vi "VPConv_SM.vi"() -> ()   [LabVIEW 2019]
uses:
  <vilib>/Utility/file.llb/Write Delimited Spreadsheet (DBL).vi
  <vilib>/Utility/file.llb/Read Delimited Spreadsheet (DBL).vi
  <vilib>/Analysis/NI_AALBase.lvlib
panel:
  out "Current State":string
  in  "Tab Control":enum32{"Mask A", "Mask B"}(tab)
  out "Intensity A":cluster{dbl[], dbl[]}[](graph)
  out "Phase A":cluster{"Ramp Pattern":dbl[], "phase out":dbl[]}(graph)
  out "Cur A":sgl
  out "Intensity B":cluster{dbl[], dbl[]}[](graph)
  out "Phase B":cluster{"Ramp Pattern":dbl[], "phase out":dbl[]}(graph)
  out "Cur B":sgl
  in  "Use Max Voltage Range for B?":bool
  in  "Save Path":path=path "C:/Users/Pubudu Wijesinghe/Desktop/VPConv"
  in  "Calib Path":path=path "C:/Users/Pubudu Wijesinghe/Desktop/Voltage Calib"
  in  "Min Cut-off":sgl=0.25
  in  "Max Cut-on":sgl=0.75
  in  "Ending Pixel":sgl=500.0
  in  "Starting Pixel":sgl=200.0
  in  "Use Max Voltage Range for A?":bool
  in  "OK":bool
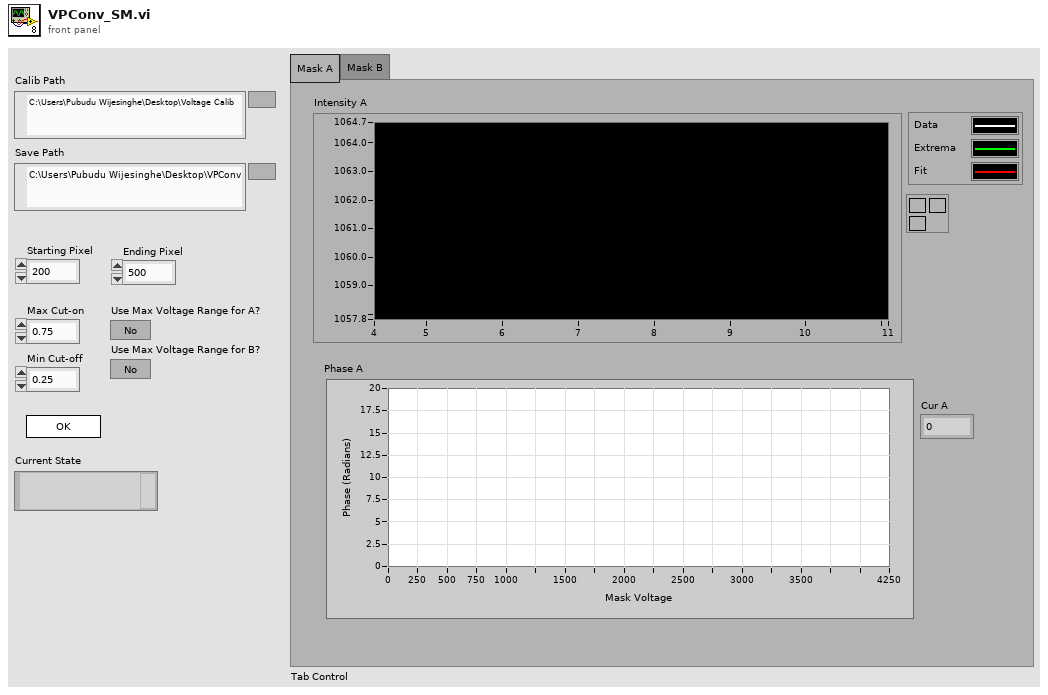
[diagram p1: front panel]
types:
  T1 = enum32{"Invalid", "Standard", "Closed", "Hidden", "Minimized", "Maximized"}
  T2 = enum32{"invalid app kind", "Development System", "Run Time System", "Student Edition", "Embedded LabVIEW", "Evaluation", "Custom"}
  T3 = cluster{"Core":cluster{"Current VI Reference":refnum<vi>, "Close Panel on Exit?":bool}, "Your Boolean data":bool, "Your string data":string, "Calib Path":path, "Save Path":path, "Starting Pixel":sgl, "Ending Pixel":sgl, "Max Cut-on":sgl, "Min Cut-off":sgl}
  T4 = cluster{"Current VI Reference":refnum<vi>, "Close Panel on Exit?":bool}
  T5 = cluster{"type":enum16{"minimum", "maximum"}, "x":i32, "y":dbl}[]
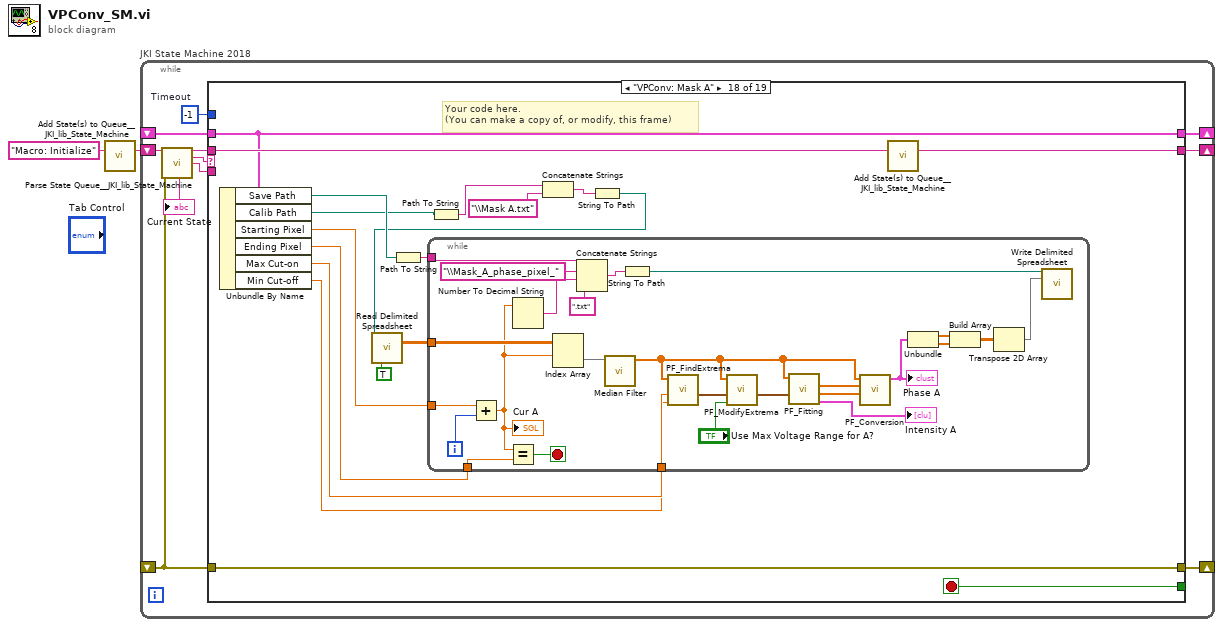
[diagram p0: block diagram]
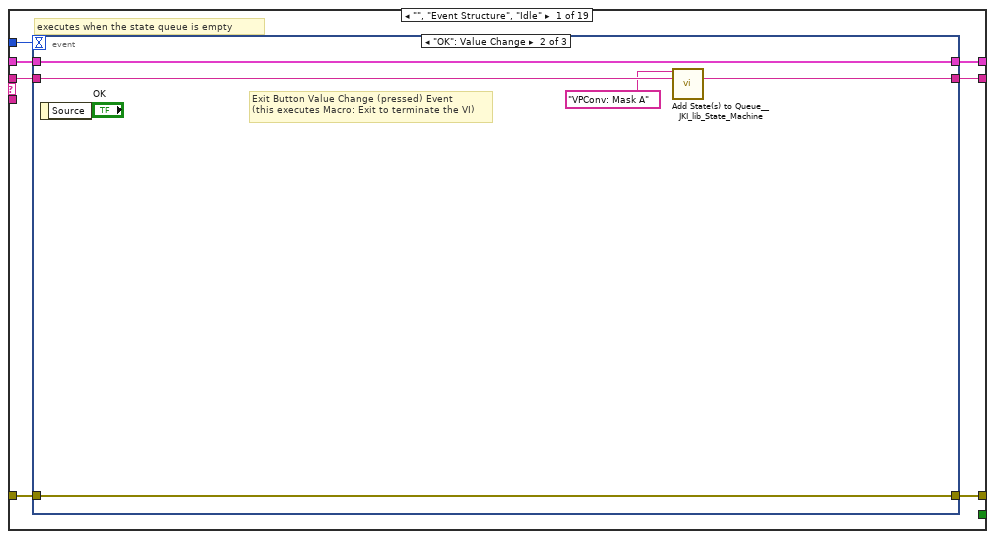
[diagram p2: hidden frame]
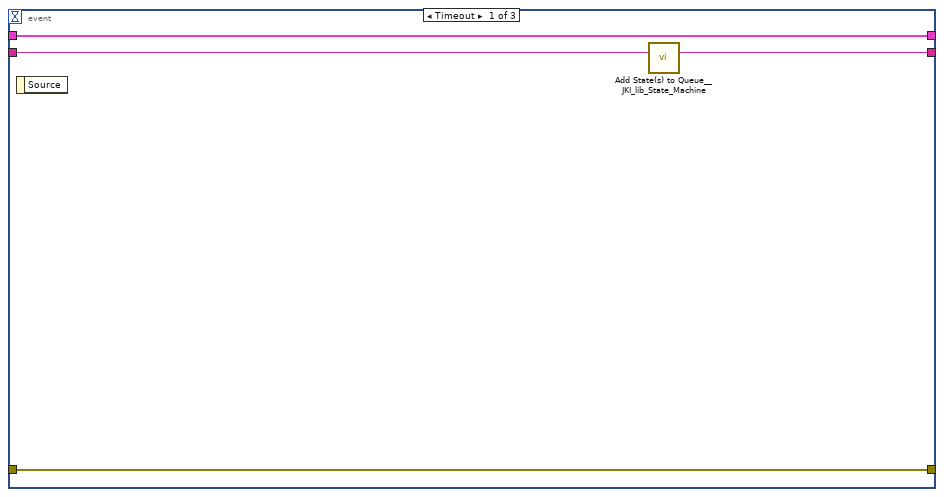
[diagram p3: hidden frame]
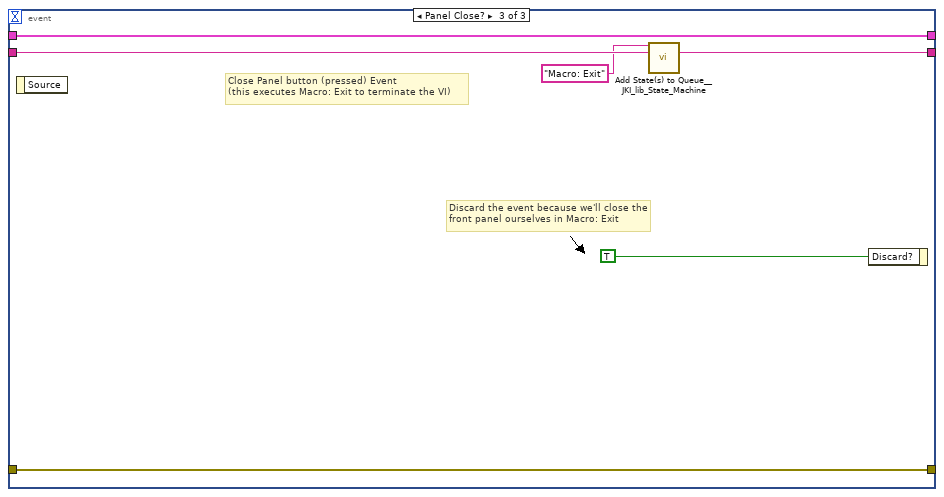
[diagram p4: hidden frame]
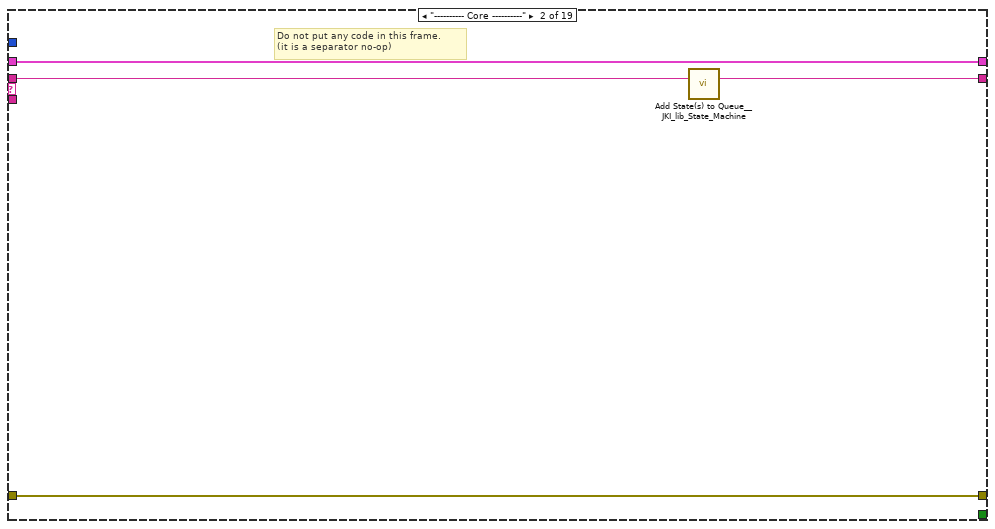
[diagram p5: hidden frame]
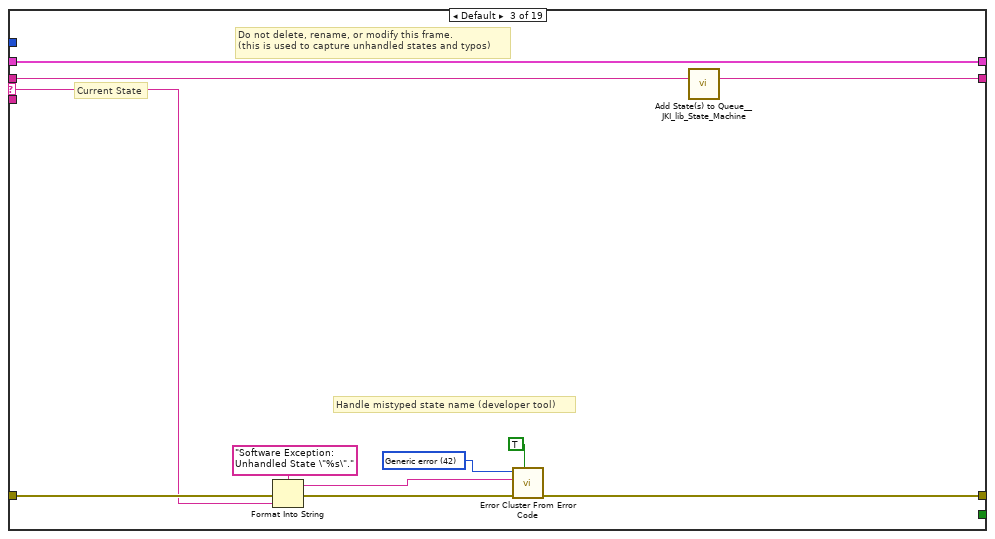
[diagram p6: hidden frame]
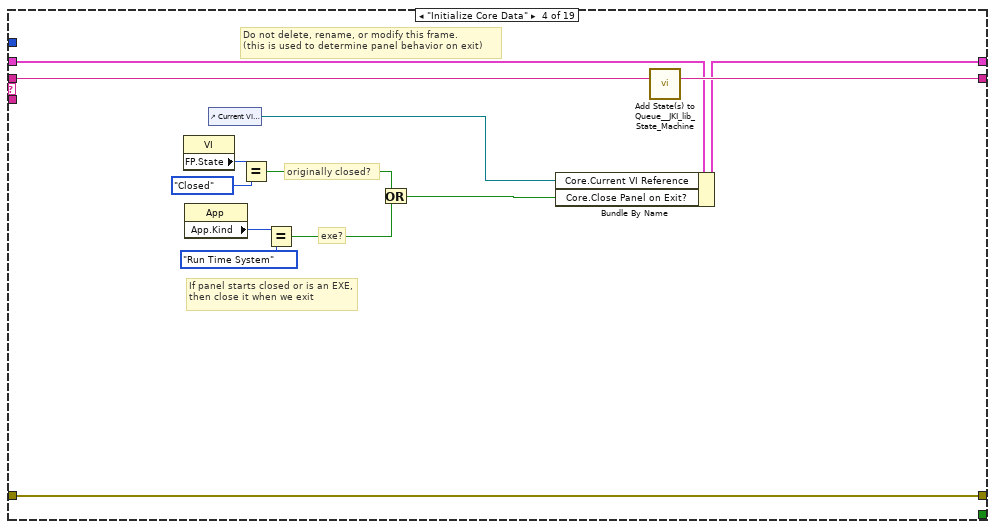
[diagram p7: hidden frame]
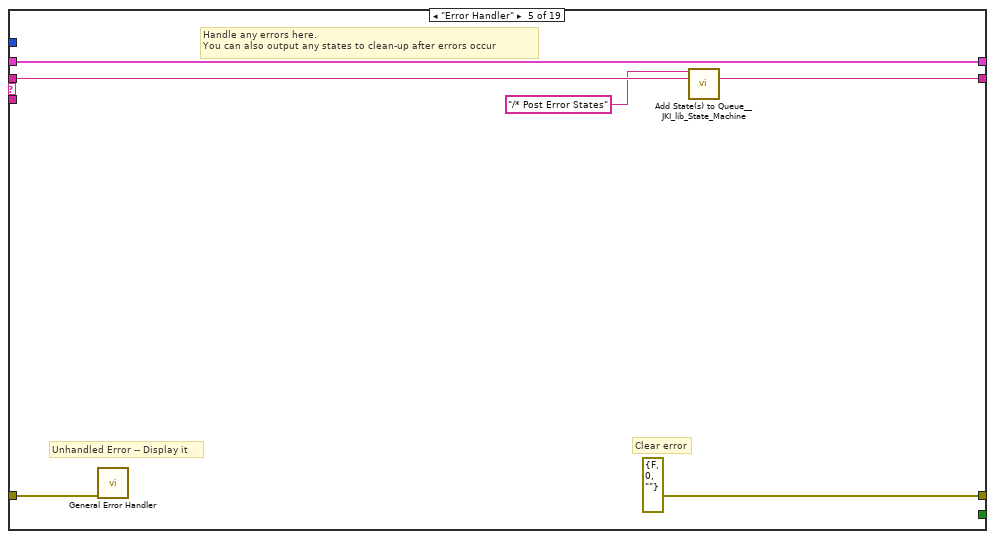
[diagram p8: hidden frame]
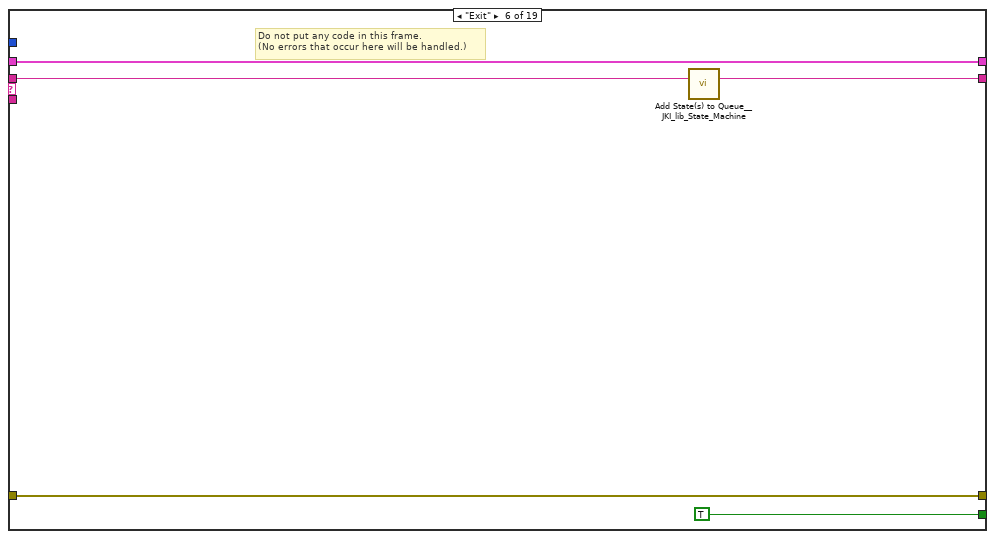
[diagram p9: hidden frame]
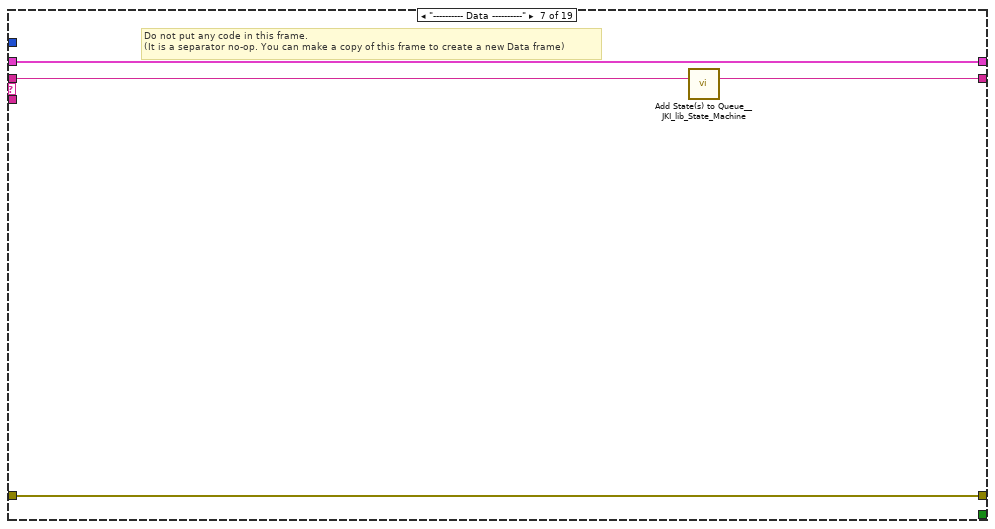
[diagram p10: hidden frame]
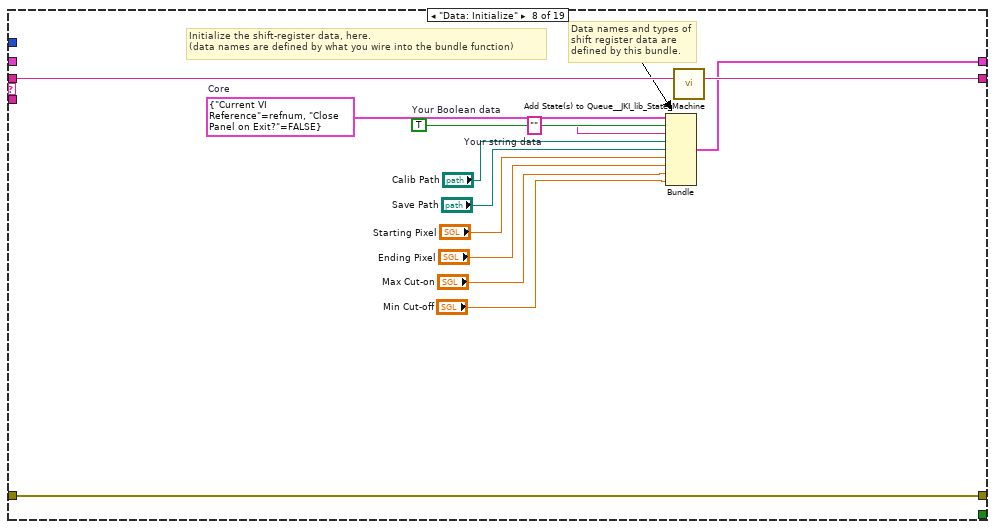
[diagram p11: hidden frame]
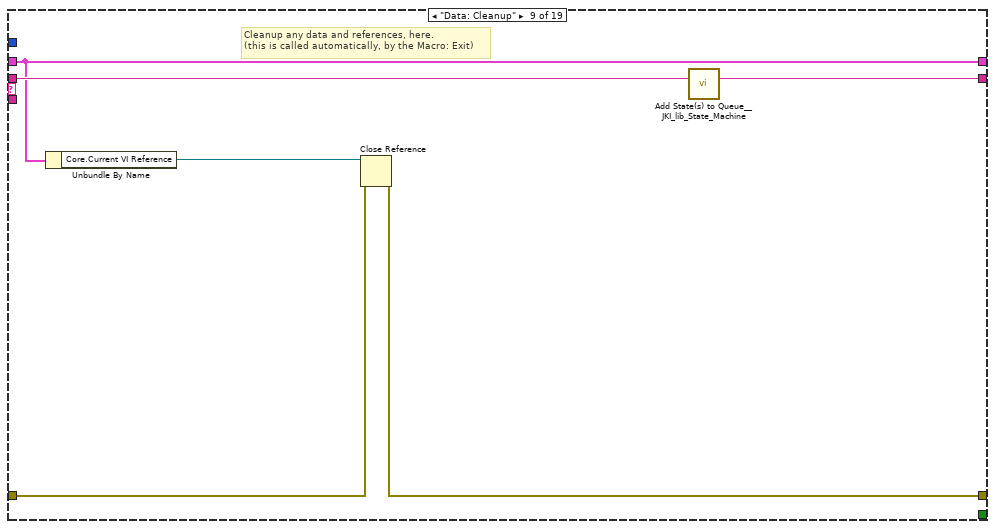
[diagram p12: hidden frame]
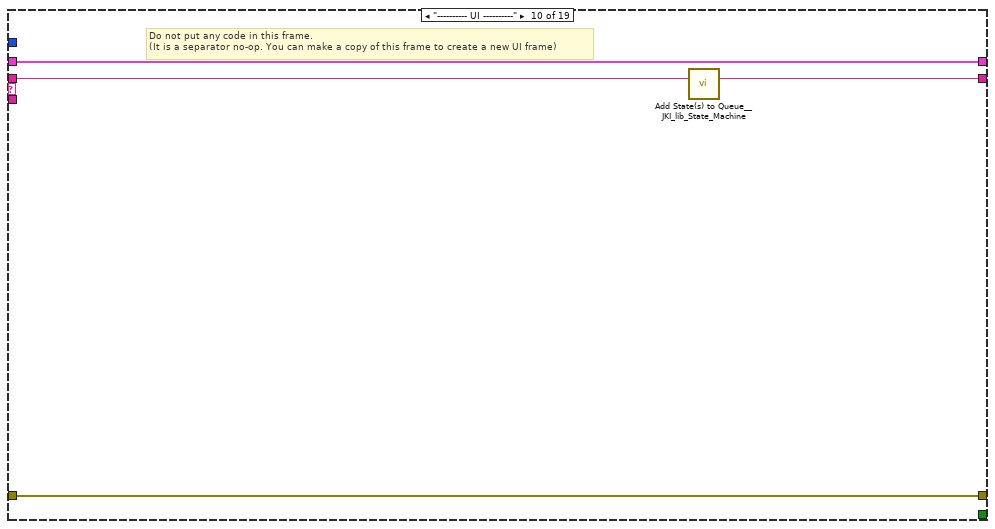
[diagram p13: hidden frame]
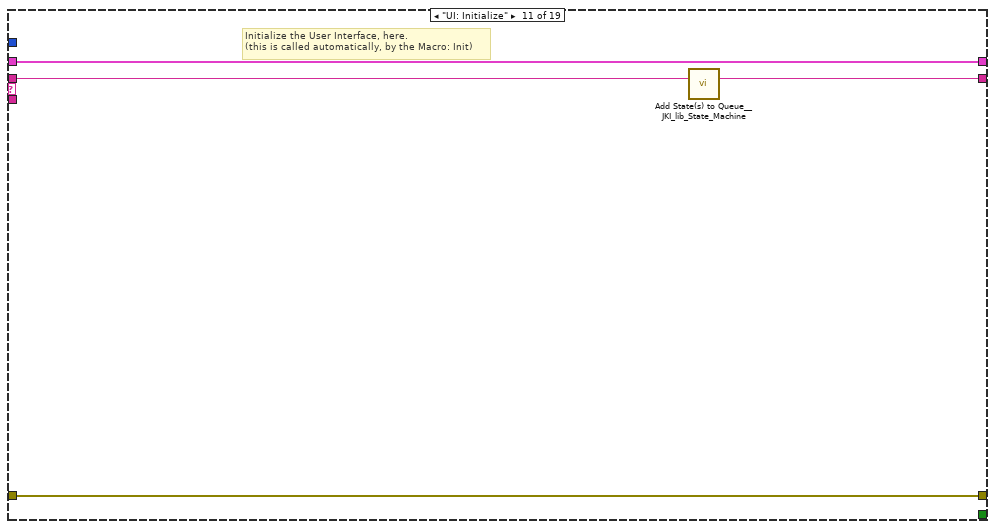
[diagram p14: hidden frame]
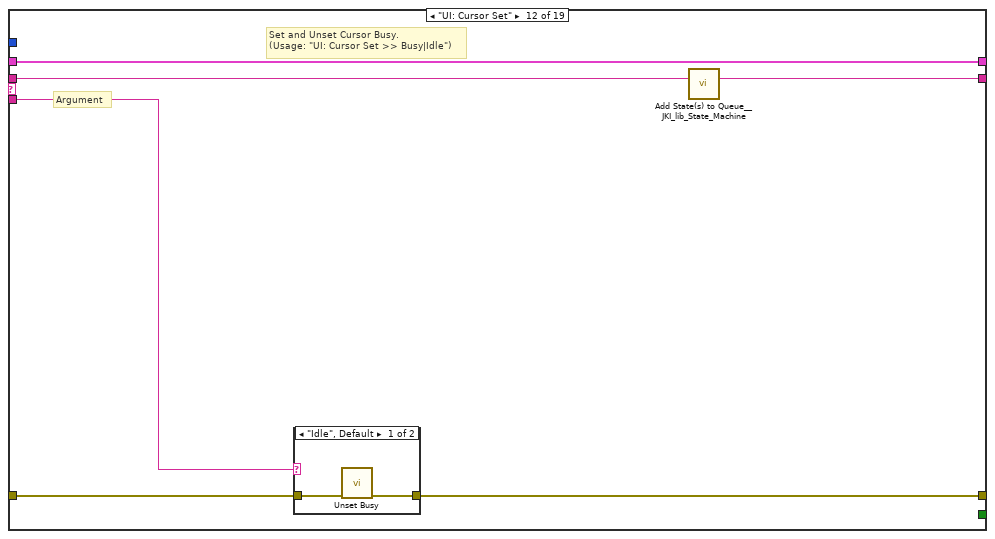
[diagram p15: hidden frame]
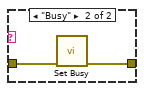
[diagram p16: hidden frame]
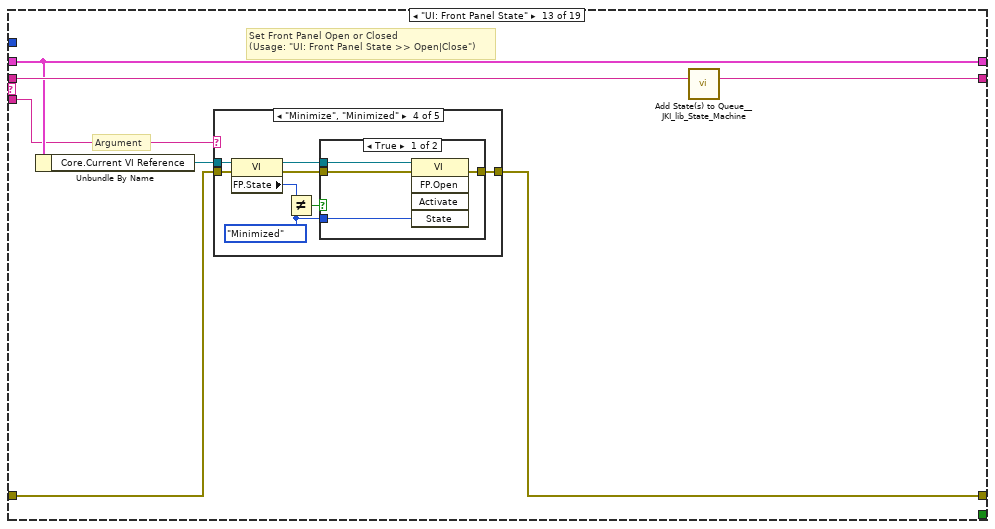
[diagram p17: hidden frame]
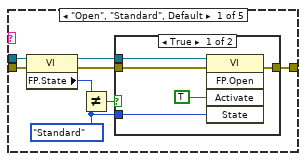
[diagram p18: hidden frame]
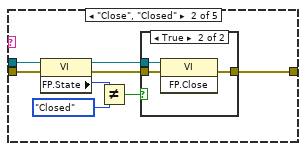
[diagram p20: hidden frame]
diagram:
  n1 = call <vilib>:"Add State(s) to Queue__JKI_lib_State_Machine.vi"("State(s) in (\"\")"="Macro: Initialize") -> ("States Out"=w2:string)  [unwired: 14 in]
  n2 = while "JKI State Machine 2018" {
    shift-right: [w6] -> _
    shift-left: _ -> [w5]
    shift-right: [w9] -> _
    shift-left: _ -> [w3]
    shift-right: [w8] -> _
    shift-left: w2 -> [w10]
    stop <- w7 stop-if-true
    w4 = -1  # Timeout
    n3 = call <vilib>:"Parse State Queue__JKI_lib_State_Machine.vi"("State Queue"=w10, "Error In (no error)"=w3) -> ("Remaining States"=w12:string, "Current State"=w13:string, "Arguments"=w11:string)  [unwired: 11 in]
    "Current State" <- w13
    n4 = case shown="\"VPConv: Mask A\"" w13 {
      selector: w13 -> [_ _ w40 _ _ _ _ _ _ _ _ _ _ _ _ _ _ _ _]
      tunnel: w12 -> [w20 w39 w44 w63 w69 w74 w78 w91 w97 w101 w105 w111 w122 w191 w196 w206 w210 w227 w271]
      tunnel: w11 -> [_ _ _ _ _ _ _ _ _ _ _ w106 w116 _ _ _ _ _ _]
      tunnel: w5 -> [w18 w36 w42 w56 w66 w72 w75 _ w92 w98 w103 w109 w118 w188 w193 w203 w207 w222 w266]
      tunnel: [w17 w37 w46 w60 errorcluster {"status"=FALSE, "code"=0, "source"=""} ("error out") w71 w76 w88 w93 w99 w102 w107 w119 w189 w194 w204 w208 w225 w269] -> w9
      tunnel: w3 -> [w16 w37 w45 w60 w65 w71 w76 w88 w94 w99 w102 w108 w120 w189 w194 w204 w208 w225 w269]
      tunnel: [w19 w38 w43 w62 w68 w73 w77 w90 w96 w100 w104 w110 w121 w190 w195 w205 w209 w226 w270] -> w8
      tunnel: [_ _ _ _ _ TRUE _ _ _ _ _ _ _ _ _ _ _ _ _] -> w7
      tunnel: [w15 w36 w42 w61 w66 w72 w75 w89 w92 w98 w103 w109 w118 w188 w193 w203 w207 w222 w266] -> w6
      tunnel: w4 -> [w14 _ _ _ _ _ _ _ _ _ _ _ _ _ _ _ _ _ _]
      frame "", "Event Structure", "Idle" {
        # "executes when the state queue is empty"
        n5 = event shown="[1] \"OK\": Value Change" {
          selector: _ -> [_ _ _]
          dyn-events: _ -> [_ _ _]
          timeout: w14 -> [_ _ _]
          tunnel: w20 -> [w24 w29 w35]
          tunnel: [w23 w28 w34] -> w19
          tunnel: w18 -> [w21 w26 w32]
          tunnel: [w22 w27 w33] -> w17
          tunnel: w16 -> [w22 w27 w33]
          tunnel: [w21 w26 w32] -> w15
          event Timeout {
            n6 = event-data() -> ()  [unwired: 1 in, 1 out]
            n7 = call <vilib>:"Add State(s) to Queue__JKI_lib_State_Machine.vi"("State(s) in (\"\")"=w24) -> ("States Out"=w23:string)  [unwired: 14 in]
          }
          event "OK": Value Change {
            # "Exit Button Value Change (pressed) Event\n(this executes Macro: Exit to terminate the VI)"
            n8 = event-data() -> ()  [unwired: 1 in, 1 out]
            n9 = call <vilib>:"Add State(s) to Queue__JKI_lib_State_Machine.vi"("State(s) in Front (\"\")"="VPConv: Mask A", "State(s) in (\"\")"=w29) -> ("States Out"=w28:string)  [unwired: 13 in]
          }
          event Panel Close? {
            # "Discard the event because we'll close the front panel ourselves in Macro: Exit"
            # "Close Panel button (pressed) Event\n(this executes Macro: Exit to terminate the VI)"
            n10 = event-data() -> ()  [unwired: 1 in, 1 out]
            n11 = call <vilib>:"Add State(s) to Queue__JKI_lib_State_Machine.vi"("State(s) in Front (\"\")"="Macro: Exit", "State(s) in (\"\")"=w35) -> ("States Out"=w34:string)  [unwired: 13 in]
            n12 = event-data("Discard?"=TRUE) -> ()  [unwired: 1 in, 1 out]
          }
        }
      }
      frame "---------- Core ----------" {
        # "Do not put any code in this frame.\n(it is a separator no-op)"
        n13 = call <vilib>:"Add State(s) to Queue__JKI_lib_State_Machine.vi"("State(s) in (\"\")"=w39) -> ("States Out"=w38:string)  [unwired: 14 in]
      }
      frame Default {
        w49 = 42 items=["No error", "Argument error", "Memory is full", "Out of zone", "End of file", "File already open", "Generic file I/O error", "File not found", "File permission error", "Disk is full", "Duplicate path", "Too many files open", "System feature not enabled", "Resource file not found", "Cannot add resource", "Resource not found", "Image not found", "Image memory error", "Pen does not exist", "Config type invalid", "Config token not found", "Config parse error", "Config memory error", "Bad external code format", "Bad external code offset", "External code not present", "Null window", "Destroy window error", "Null menu", "Print aborted", "Bad print record", "Print driver error", "Windows error during printing", "Memory error during printing", "Print dialog error", "Generic print error", "Invalid device refnum", "Device not found", "Device parameter error", "Device unit error", "Cannot open device", "Device call aborted", "Generic error", "Cancelled by user", "Object ID too low", "Object ID too high", "Object not in heap", "Unknown heap", "Unknown object (invalid DefProc)", "Unknown object (DefProc not in table)", "Message out of range", "Invalid (null) method", "Unknown message", "Manager call not supported", "Bad address", "Network operation in progress", "Network operation timed out", "Connection is busy", "Network attribute not supported", "Network error", "Address in use", "System out of memory", "Connection aborted", "Connection refused", "Not connected", "Already connected", "Connection closed", "Initialization error (interapplication manager)", "Bad occurrence", "Wait on unbound occurrence handler", "Occurrence queue overflow", "Datalog type conflict", "Unused", "Unrecognized type (interapplication manager)", "Memory corrupt", "Failed to make temporary DLL", "Old CIN version", "Drag socket not found", "Failed to load drop-object", "Failed to register OLE object", "Failed to release OLE object", "Format specifier type mismatch", "Unknown format specifier", "Too few format specifiers", "Too many format specifiers", "Scan failed", "Newer CIN version", "Error converting to variant", "Runtime menu error", "Password tampered", "Variant attribute not found", "Incompatible variant data type", "Event data is not available", "Event Store is not present", "Occurrence is not found", "Event Queue is not created", "Event info is not available", "Refnum passed is NULL", "Error retrieving Class GUID", "Error retrieving CoClass GUID", "Error retrieving TypeLib GUID.", "Bad built application magic bytes.", "Specific driver is different from the specific driver associated with the Logical Name.", "There is no session opened to the class driver.", "Max Error", "MAX - Error with config objects", "MAX - Error loading configuration", "MAX - Group not supported"]
        # "Current State"
        # "Do not delete, rename, or modify this frame.\n(this is used to capture unhandled states and typos)"
        # "Handle mistyped state name (developer tool)"
        n14 = Format Into String(format string="Software Exception: Unhandled State \"%s\"." ("message"), error in=w45, w40) -> (resulting string=w48:string, error out=w47:errorcluster)  [unwired: 1 in]
        n15 = call <vilib>:"Error Cluster From Error Code.vi"("show call chain? (False)"=TRUE, "error in (no error)"=w47, "error message (\"\")"=w48, "error code (0)"=w49) -> ("error out"=w46:errorcluster)  [unwired: 5 in]
        n16 = call <vilib>:"Add State(s) to Queue__JKI_lib_State_Machine.vi"("State(s) in (\"\")"=w44) -> ("States Out"=w43:string)  [unwired: 14 in]
      }
      frame "Initialize Core Data" {
        # "Do not delete, rename, or modify this frame.\n(this is used to determine panel behavior on exit)"
        # "originally closed?"
        # "exe?"
        # "If panel starts closed or is an EXE, then close it when we exit"
        n17 = property class="VI"() -> ("FP.State"=w53:T1)  [unwired: 2 in, 2 out]
        n18 = property class="App"() -> ("App.Kind"=w59:T2)  [unwired: 2 in, 2 out]
        n19 = control-ref of="Current VI Reference"() -> (w54:refnum<vi>)
        n20 = Equal?(x=w53, y=T1."Closed" ("Front Panel Window:State")) -> (x = y?=w51:bool)
        n21 = Equal?(x=w59, y=T2."Run Time System" ("Application:Kind")) -> (x = y?=w57:bool)
        n22 = Or(x=w51, y=w57) -> (x .or. y?=w55:bool)
        n23 = Bundle By Name(cluster=w56, "Core.Current VI Reference"=w54, "Core.Close Panel on Exit?"=w55) -> (w61:T3)
        n24 = call <vilib>:"Add State(s) to Queue__JKI_lib_State_Machine.vi"("State(s) in (\"\")"=w63) -> ("States Out"=w62:string)  [unwired: 14 in]
      }
      frame "Error Handler" {
        # "Unhandled Error -- Display it"
        # "Handle any errors here.\nYou can also output any states to clean-up after errors occur"
        # "Clear error"
        n25 = call <vilib>:"General Error Handler.vi"("error in (no error)"=w65) -> ()  [unwired: 10 in, 5 out]
        n26 = call <vilib>:"Add State(s) to Queue__JKI_lib_State_Machine.vi"("State(s) in Front (\"\")"="/* Post Error States", "State(s) in (\"\")"=w69) -> ("States Out"=w68:string)  [unwired: 13 in]
      }
      frame "Exit" {
        # "Do not put any code in this frame.\n(No errors that occur here will be handled.)"
        n27 = call <vilib>:"Add State(s) to Queue__JKI_lib_State_Machine.vi"("State(s) in (\"\")"=w74) -> ("States Out"=w73:string)  [unwired: 14 in]
      }
      frame "---------- Data ----------" {
        # "Do not put any code in this frame.\n(It is a separator no-op. You can make a copy of this frame to create a new Data frame)"
        n28 = call <vilib>:"Add State(s) to Queue__JKI_lib_State_Machine.vi"("State(s) in (\"\")"=w78) -> ("States Out"=w77:string)  [unwired: 14 in]
      }
      frame "Data: Initialize" {
        w85 = T4 {"Current VI Reference"=refnum, "Close Panel on Exit?"=FALSE}  # Core
        w87 = TRUE  # Your Boolean data
        w86 = ""  # Your string data
        # "Data names and types of shift register data are defined by this bundle."
        # "Initialize the shift-register data, here.\n(data names are defined by what you wire into the bundle function)"
        n29 = Bundle("Core"=w85, "Your Boolean data"=w87, "Your string data"=w86, "Calib Path"="Calib Path", "Save Path"="Save Path", "Starting Pixel"="Starting Pixel", "Ending Pixel"="Ending Pixel", "Max Cut-on"="Max Cut-on", "Min Cut-off"="Min Cut-off") -> (w89:T3)  [unwired: 1 in]
        n30 = call <vilib>:"Add State(s) to Queue__JKI_lib_State_Machine.vi"("State(s) in (\"\")"=w91) -> ("States Out"=w90:string)  [unwired: 14 in]
      }
      frame "Data: Cleanup" {
        # "Cleanup any data and references, here.\n(this is called automatically, by the Macro: Exit)"
        n31 = Unbundle By Name(w92) -> ("Core.Current VI Reference"=w95:refnum<vi>)
        n32 = Close Reference(reference=w95, error in (no error)=w94) -> (error out=w93:errorcluster)
        n33 = call <vilib>:"Add State(s) to Queue__JKI_lib_State_Machine.vi"("State(s) in (\"\")"=w97) -> ("States Out"=w96:string)  [unwired: 14 in]
      }
      frame "---------- UI ----------" {
        # "Do not put any code in this frame.\n(It is a separator no-op. You can make a copy of this frame to create a new UI frame)"
        n34 = call <vilib>:"Add State(s) to Queue__JKI_lib_State_Machine.vi"("State(s) in (\"\")"=w101) -> ("States Out"=w100:string)  [unwired: 14 in]
      }
      frame "UI: Initialize" {
        # "Initialize the User Interface, here.\n(this is called automatically, by the Macro: Init)"
        n35 = call <vilib>:"Add State(s) to Queue__JKI_lib_State_Machine.vi"("State(s) in (\"\")"=w105) -> ("States Out"=w104:string)  [unwired: 14 in]
      }
      frame "UI: Cursor Set" {
        # "Argument"
        # "Set and Unset Cursor Busy.\n(Usage: \"UI: Cursor Set >> Busy|Idle\")"
        n36 = case shown="\"Idle\", Default" w106 {
          tunnel: w108 -> [w113 w115]
          tunnel: [w112 w114] -> w107
          frame "Idle", Default {
            n37 = call <vilib>:"Unset Busy.vi"("error in (no error)"=w113) -> ("error out"=w112:errorcluster)  [unwired: 10 in]
          }
          frame "Busy" {
            n38 = call <vilib>:"Set Busy.vi"("error in (no error)"=w115) -> ("error out"=w114:errorcluster)  [unwired: 9 in, 1 out]
          }
        }
        n39 = call <vilib>:"Add State(s) to Queue__JKI_lib_State_Machine.vi"("State(s) in (\"\")"=w111) -> ("States Out"=w110:string)  [unwired: 14 in]
      }
      frame "UI: Front Panel State" {
        # "Argument"
        # "Set Front Panel Open or Closed\n(Usage: \"UI: Front Panel State >> Open|Close\")"
        n40 = Unbundle By Name(w118) -> ("Core.Current VI Reference"=w117:refnum<vi>)
        n41 = case shown="\"Minimize\", \"Minimized\"" w116 {
          tunnel: w120 -> [w128 w143 w154 w167 w180]
          tunnel: [w130 w144 w156 w169 w182] -> w119
          tunnel: w117 -> [w129 w141 w155 w168 w181]
          frame "Open", "Standard", Default {
            w123 = T1."Standard" ("State")
            n42 = property class="VI"(reference=w129, error in=w128) -> (reference out=w126:refnum<vi>, error out=w127:errorcluster, "FP.State"=w125:T1)
            n43 = Not Equal?(x=w125, y=w123) -> (x != y?=w124:bool)
            n44 = case shown="True" w124 {
              tunnel: [w134 w136] -> w130
              tunnel: w127 -> [w133 w136]
              tunnel: w126 -> [w132 _]
              tunnel: w123 -> [w131 _]
              frame True {
                n45 = invoke class="VI" method="FP.Open"(reference=w132, error in=w133, "Activate"=TRUE, "State"=w131) -> (error out=w134:errorcluster)  [unwired: 1 in, 4 out]
              }
              frame False {
              }
            }
          }
          frame "Close", "Closed" {
            n46 = property class="VI"(reference=w141, error in=w143) -> (reference out=w140:refnum<vi>, error out=w142:errorcluster, "FP.State"=w138:T1)
            n47 = Not Equal?(x=w138, y=T1."Closed" ("Front Panel Window:State")) -> (x != y?=w137:bool)
            n48 = case shown="True" w137 {
              tunnel: [w145 w148] -> w144
              tunnel: w142 -> [w145 w147]
              tunnel: w140 -> [_ w146]
              frame False {
              }
              frame True {
                n49 = invoke class="VI" method="FP.Close"(reference=w146, error in=w147) -> (error out=w148:errorcluster)  [unwired: 1 in, 2 out]
              }
            }
          }
          frame "Hidden", "Hide" {
            w149 = T1."Hidden" ("State")
            n50 = property class="VI"(reference=w155, error in=w154) -> (reference out=w152:refnum<vi>, error out=w153:errorcluster, "FP.State"=w151:T1)
            n51 = Not Equal?(x=w151, y=w149) -> (x != y?=w150:bool)
            n52 = case shown="True" w150 {
              tunnel: [w160 w161] -> w156
              tunnel: w153 -> [w159 w161]
              tunnel: w152 -> [w158 _]
              tunnel: w149 -> [w157 _]
              frame True {
                n53 = invoke class="VI" method="FP.Open"(reference=w158, error in=w159, "State"=w157) -> (error out=w160:errorcluster)  [unwired: 2 in, 4 out]
              }
              frame False {
              }
            }
          }
          frame "Minimize", "Minimized" {
            w162 = T1."Minimized" ("State")
            n54 = property class="VI"(reference=w168, error in=w167) -> (reference out=w165:refnum<vi>, error out=w166:errorcluster, "FP.State"=w164:T1)
            n55 = Not Equal?(x=w164, y=w162) -> (x != y?=w163:bool)
            n56 = case shown="True" w163 {
              tunnel: [w173 w174] -> w169
              tunnel: w166 -> [w172 w174]
              tunnel: w165 -> [w171 _]
              tunnel: w162 -> [w170 _]
              frame True {
                n57 = invoke class="VI" method="FP.Open"(reference=w171, error in=w172, "State"=w170) -> (error out=w173:errorcluster)  [unwired: 2 in, 4 out]
              }
              frame False {
              }
            }
          }
          frame "Maximize", "Maximized" {
            w175 = T1."Maximized" ("State")
            n58 = property class="VI"(reference=w181, error in=w180) -> (reference out=w178:refnum<vi>, error out=w179:errorcluster, "FP.State"=w177:T1)
            n59 = Not Equal?(x=w177, y=w175) -> (x != y?=w176:bool)
            n60 = case shown="True" w176 {
              tunnel: [w186 w187] -> w182
              tunnel: w179 -> [w185 w187]
              tunnel: w178 -> [w184 _]
              tunnel: w175 -> [w183 _]
              frame True {
                n61 = invoke class="VI" method="FP.Open"(reference=w184, error in=w185, "State"=w183) -> (error out=w186:errorcluster)  [unwired: 2 in, 4 out]
              }
              frame False {
              }
            }
          }
        }
        n62 = call <vilib>:"Add State(s) to Queue__JKI_lib_State_Machine.vi"("State(s) in (\"\")"=w122) -> ("States Out"=w121:string)  [unwired: 14 in]
      }
      frame "---------- Macro ----------" {
        # "Do not put any code in this frame.\n(It is a separator no-op. You can make a copy of this frame to create a new Macro frame)"
        n63 = call <vilib>:"Add State(s) to Queue__JKI_lib_State_Machine.vi"("State(s) in (\"\")"=w191) -> ("States Out"=w190:string)  [unwired: 14 in]
      }
      frame "Macro: Initialize" {
        w192 = "Data: Initialize\nInitialize Core Data\nUI: Initialize\nUI: Front Panel State >> Open"  # Data: Initialize Initialize Core Data UI: Initialize UI: Front Panel State >> Open
        # "Initialization Macro\n(This is called once, when the VI starts)"
        n64 = call <vilib>:"Add State(s) to Queue__JKI_lib_State_Machine.vi"("State(s) in Front (\"\")"=w192, "State(s) in (\"\")"=w196) -> ("States Out"=w195:string)  [unwired: 13 in]
      }
      frame "Macro: Exit" {
        # "Exit Macro\n(This is called once, when the VI exits)"
        n65 = Unbundle By Name(w203) -> ("Core.Close Panel on Exit?"=w202:bool)
        n66 = Select(t="UI: Front Panel State >> Close", s=w202, f="") -> (s? t:f=w199:string)
        n67 = call <vilib>:"Add State(s) to Queue__JKI_lib_State_Machine.vi"("State(s) in (\"\")"=w199, "State(s) at Back (\"\")"="Data: Cleanup\nExit") -> ("States Out"=w197:string)  [unwired: 13 in]
        n68 = call <vilib>:"Add State(s) to Queue__JKI_lib_State_Machine.vi"("State(s) in Front (\"\")"=w197, "State(s) in (\"\")"=w206) -> ("States Out"=w205:string)  [unwired: 13 in]
      }
      frame "---------- VPConv ----------" {
        # "Template Separator\n(You can make a copy of, or modify, this frame)"
        n69 = call <vilib>:"Add State(s) to Queue__JKI_lib_State_Machine.vi"("State(s) in (\"\")"=w210) -> ("States Out"=w209:string)  [unwired: 14 in]
      }
      frame "VPConv: Mask A" {
        # "Your code here.\n(You can make a copy of, or modify, this frame)"
        n70 = Unbundle By Name(w222) -> ("Save Path"=w221:path, "Calib Path"=w212:path, "Starting Pixel"=w219:sgl, "Ending Pixel"=w218:sgl, "Max Cut-on"=w217:sgl, "Min Cut-off"=w216:sgl)
        n71 = Path To String(path=w221) -> (string=w220:string)
        n72 = Path To String(path=w212) -> (string=w215:string)
        n73 = Concatenate Strings(w215, "\\Mask A.txt" ("string")) -> (w213:string)
        n74 = String To Path(string=w213) -> (path=w211:path)
        n75 = call-poly <vilib>:"Read Delimited Spreadsheet.vi"("file path (dialog if empty)"=w211, "transpose? (F)"=TRUE) -> ("all rows"=w223:dbl[][])  [unwired: 8 in, 5 out]
        n76 = while {
          tunnel: w223 -> [w248]
          tunnel: w220 -> [w235]
          tunnel: w219 -> [w234]
          tunnel: w218 -> [w233]
          tunnel: w217 -> [w232]
          tunnel: w216 -> [w231]
          i -> [w246]
          stop <- w247 stop-if-true
          n77 = Add(x=w234, y=w246) -> (x+y=w243:sgl)
          "Cur A" <- w243
          n78 = Equal?(x=w243, y=w233) -> (x = y?=w247:bool)
          n79 = Number To Decimal String(number=w243) -> (decimal integer string=w244:string)  [unwired: 1 in]
          n80 = Index Array(array=w248, index (row)=w243) -> (element=w229:dbl[])  [unwired: 1 in]
          n81 = Concatenate Strings(w235, "\\Mask_A_phase_pixel_", w244, ".txt" ("string")) -> (w242:string)
          n82 = call <vilib>:"Median Filter.vi"("X"=w229) -> ("Filtered X"=w228:dbl[])  [unwired: 9 in, 1 out]
          n83 = String To Path(string=w242) -> (path=w236:path)
          n84 = call "PF_FindExtrema.vi"("Min Cut-off"=w231, "Max Cut-on"=w232, "Intensity Array"=w228) -> ("Extrema Array"=w254:T5)  [unwired: 7 in]
          n85 = call "PF_ModifyExtrema.vi"("Max Voltage Range?"="Use Max Voltage Range for A?", "Extremas Array In"=w254, "Intensity Array"=w228) -> ("Extremas Array Out"=w252:T5)  [unwired: 8 in]
          n86 = call "PF_Fitting.vi"("Extrema Array"=w252, "Intensity Array"=w228) -> ("Intensity"=→"Intensity A":cluster{dbl[], dbl[]}[], "yFit"=w250:dbl[], "xFit"=w251:dbl[])  [unwired: 6 in]
          n87 = call "PF_Conversion.vi"("Intensity"=w228, "xFit"=w251, "yFit"=w250) -> ("Phase"=w238:cluster{"Ramp Pattern":dbl[], "phase out":dbl[]})  [unwired: 7 in]
          "Phase A" <- w238
          n88 = Unbundle(w238) -> ("Ramp Pattern"=w241:dbl[], "phase out"=w240:dbl[])
          n89 = Build Array(w241, w240) -> (w239:dbl[][])
          n90 = Transpose 2D Array(2D array=w239) -> (transposed array=w237:dbl[][])
          n91 = call-poly <vilib>:"Write Delimited Spreadsheet.vi"("file path (dialog if empty)"=w236, "2D data"=w237) -> ()  [unwired: 12 in, 2 out]
        }
        n92 = call <vilib>:"Add State(s) to Queue__JKI_lib_State_Machine.vi"("State(s) in (\"\")"=w227) -> ("States Out"=w226:string)  [unwired: 14 in]
      }
      frame "VPConv: Mask B" {
        n93 = Unbundle By Name(w266) -> ("Save Path"=w265:path, "Calib Path"=w259:path, "Starting Pixel"=w263:sgl, "Ending Pixel"=w262:sgl, "Max Cut-on"=w261:sgl, "Min Cut-off"=w260:sgl)
        n94 = Path To String(path=w259) -> (string=w258:string)
        n95 = Path To String(path=w265) -> (string=w264:string)
        n96 = Concatenate Strings(w258, "\\Mask B.txt" ("string")) -> (w256:string)
        n97 = String To Path(string=w256) -> (path=w255:path)
        n98 = call-poly <vilib>:"Read Delimited Spreadsheet.vi"("file path (dialog if empty)"=w255, "transpose? (F)"=TRUE) -> ("all rows"=w267:dbl[][])  [unwired: 8 in, 5 out]
        n99 = while {
          tunnel: w267 -> [w291]
          tunnel: w264 -> [w277]
          tunnel: w263 -> [w276]
          tunnel: w262 -> [w275]
          tunnel: w261 -> [w274]
          tunnel: w260 -> [w273]
          i -> [w288]
          stop <- w289 stop-if-true
          n100 = Add(x=w276, y=w288) -> (x+y=w285:sgl)
          "Cur B" <- w285
          n101 = Equal?(x=w285, y=w275) -> (x = y?=w289:bool)
          n102 = Number To Decimal String(number=w285) -> (decimal integer string=w286:string)  [unwired: 1 in]
          n103 = Index Array(array=w291, index (row)=w285) -> (element=w290:dbl[])  [unwired: 1 in]
          n104 = Concatenate Strings(w277, "\\Mask_B_phase_pixel_", w286, ".txt" ("string")) -> (w284:string)
          n105 = String To Path(string=w284) -> (path=w278:path)
          n106 = call "PF_FindExtrema.vi"("Min Cut-off"=w273, "Max Cut-on"=w274, "Intensity Array"=w290) -> ("Extrema Array"=w297:T5)  [unwired: 7 in]
          n107 = call "PF_ModifyExtrema.vi"("Max Voltage Range?"="Use Max Voltage Range for B?", "Extremas Array In"=w297, "Intensity Array"=w290) -> ("Extremas Array Out"=w295:T5)  [unwired: 8 in]
          n108 = call "PF_Fitting.vi"("Extrema Array"=w295, "Intensity Array"=w290) -> ("Intensity"=→"Intensity B":cluster{dbl[], dbl[]}[], "yFit"=w293:dbl[], "xFit"=w294:dbl[])  [unwired: 6 in]
          n109 = call "PF_Conversion.vi"("Intensity"=w290, "xFit"=w294, "yFit"=w293) -> ("Phase"=w280:cluster{"Ramp Pattern":dbl[], "phase out":dbl[]})  [unwired: 7 in]
          "Phase B" <- w280
          n110 = Unbundle(w280) -> ("Ramp Pattern"=w283:dbl[], "phase out"=w282:dbl[])
          n111 = Build Array(w283, w282) -> (w281:dbl[][])
          n112 = Transpose 2D Array(2D array=w281) -> (transposed array=w279:dbl[][])
          n113 = call-poly <vilib>:"Write Delimited Spreadsheet.vi"("file path (dialog if empty)"=w278, "2D data"=w279) -> ()  [unwired: 12 in, 2 out]
        }
        n114 = call <vilib>:"Add State(s) to Queue__JKI_lib_State_Machine.vi"("State(s) in (\"\")"=w271) -> ("States Out"=w270:string)  [unwired: 14 in]
      }
    }
  }
